vi "Add Dynamic Waveform.vi"(8 "error in":errorcluster, 11 "Node Ptr":T1 format="%.0x") -> (0 "error out":errorcluster, 3 "Node Ptr out":T1=18446744073709551615 format="%.0x")   [LabVIEW 2026]
uses:
  <vilib>/NI/VeriStand Custom Device Serialization/System Explorer Action.ctl
  C:/dev/cd20_main/Source/niveristand-custom-device-wizard/ProjectTemplate/Source/NI VeriStand/Custom Device Express/Custom Device/NationalInstruments.Veristand.Sample.dll
  NationalInstruments.Veristand.Sample.dll
  <vilib>/NI VeriStand/Custom Device API/Custom Device Item Ref.ctl
  <vilib>/NI VeriStand/Custom Device API/Custom Device API.lvlib
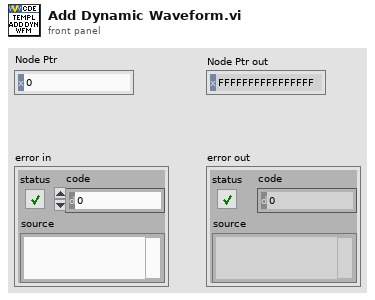
[diagram p1: front panel]
types:
  T1 = typedef "Custom Device API.lvlib/Custom Device Item Ref.ctl" = u64
  T2 = typedef "Custom Device Serialization.lvlib/System Explorer Action.ctl" = u16
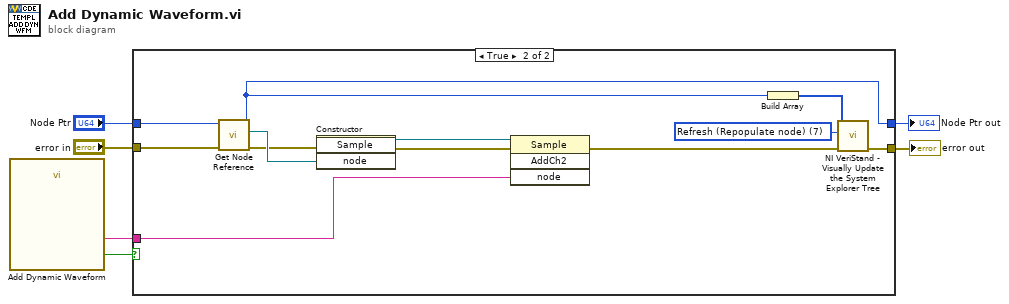
[diagram p0: block diagram]
diagram:
  n1 = call "Add Dynamic Waveform"() -> ("Waveform Name"=w2:string, "Add"=w1:bool)  [unwired: 17 in, 1 out]
  n2 = case shown="True" w1 {
    tunnel: "Node Ptr" -> [w8 w20]
    tunnel: "error in" -> [w7 w19]
    tunnel: [w8 w18] -> w4
    tunnel: [w7 w17] -> w3
    tunnel: w2 -> [_ w9]
    frame False {
    }
    frame True {
      w12 = T2 7 items=["Refresh (Add)"=5, "Refresh (Repopulate node)"=7] ("Action")
      n3 = call "Get Node Reference.vi"("error in"=w19, "Node Ptr"=w20) -> ("error out"=w11:errorcluster, "BaseNodeType"=w15:refnum<k24>, "Node Ptr"=w18:T1)  [unwired: 6 in, 1 out]
      n4 = constructor class="Sample" ("ParentConstructor")(error in=w11, "node"=w15) -> (reference out=w16:refnum<k24>, error out=w10:errorcluster)  [unwired: 2 in, 2 out]
      n5 = invoke on="AddMethodInvokeNode" class="Sample" method="AddCh2"(reference=w16, error in=w10, "node"=w9) -> (error out=w14:errorcluster)  [unwired: 1 in, 3 out]
      n6 = Build Array(w18) -> (w13:T1[])
      n7 = call <vilib>:"NI VeriStand - Visually Update the System Explorer Tree.vi"("error in (no error)"=w14, "Action"=w12, "Node IDs"=w13) -> ("error out"=w17:errorcluster)  [unwired: 8 in]
    }
  }
  "Node Ptr out" <- w4
  "error out" <- w3
